vi "Clear Map.vi"(8 "error in (no error)":errorcluster, 11 "FormulaG App in":refnum<class "FormulaG App.lvclass">) -> (0 "error out":errorcluster, 3 "FormulaG App out":refnum<class "FormulaG App.lvclass">)   [LabVIEW 2024, in "FormulaG.lvlib" / "FormulaG App.lvclass"]
uses:
  FormulaG App.lvclass
  FormulaG App.lvclass/FormulaG App.ctl
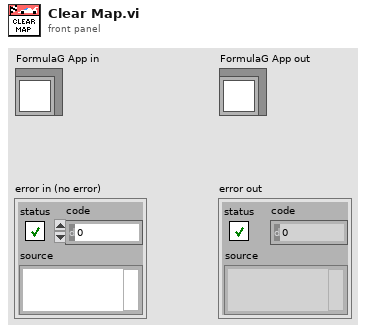
[diagram p1: front panel]
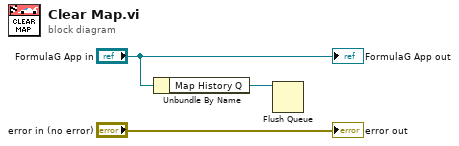
[diagram p0: block diagram]
diagram:
  n1 = Unbundle By Name("FormulaG App in") -> ("Map History Q"=w1:refnum<queue>)
  n2 = Flush Queue(queue=w1) -> ()  [unwired: 1 in, 3 out]
  "error out" <- "error in (no error)"
  "FormulaG App out" <- "FormulaG App in"
